vi "Trajectory_Execution_EXECUTE_REVERSE.vi"(5 "Track Width FT":dbl, 6 "RamseteEnable":bool=TRUE, 7 "Max Speed\nFT/SEC":dbl, 8 "Init":bool, 9 "Gyro Continous\n (inc counterclockwise)":dbl, 10 "Right Distance":dbl, 11 "Left Distance":dbl) -> (0 "AtReference":bool, 1 "Right Speed Target":dbl, 2 "Left Speed Target":dbl, 3 "outRAMSETE (SI)":T5={"B"=2.0, "Zeta"=0.7, "poseTolerance"={"TRANSLATION"={"X"=0.0, "Y"=0.0}, "ROTATION"={"VALUE"=0.0, "COS"=1.0, "SIN"=0.0}}, "poseError"={"TRANSLATION"={"X"=0.0, "Y"=0.0}, "ROTATION"={"VALUE"=0.0, "COS"=1.0, "SIN"=0.0}}, "Enabled"=TRUE} {"poseError"."ROTATION"."SIN" format="%13.4f"; "poseError"."ROTATION"."COS" format="%13.4f"; "poseError"."ROTATION"."VALUE" format="%13.4f"; "poseError"."TRANSLATION"."Y" format="%14.3f"; "poseError"."TRANSLATION"."X" format="%14.3f"; "poseTolerance"."ROTATION"."SIN" format="%13.4f"; "poseTolerance"."ROTATION"."COS" format="%13.4f"; "poseTolerance"."ROTATION"."VALUE" format="%13.4f"; "poseTolerance"."TRANSLATION"."Y" format="%14.3f"; "poseTolerance"."TRANSLATION"."X" format="%14.3f"; "Zeta" format="%12.3f"; "B" format="%12.3f"}, 4 "OutputTRAJ_STATE (SI)":T1={"TimeSeconds"=0.0, "Velocity"=0.0, "Acceleration"=0.0, "POSE"={"TRANSLATION"={"X"=0.0, "Y"=0.0}, "ROTATION"={"VALUE"=0.0, "COS"=1.0, "SIN"=0.0}}, "Curvature"=0.0} {"POSE"."ROTATION"."SIN" format="%13.4f"; "POSE"."ROTATION"."COS" format="%13.4f"; "POSE"."ROTATION"."VALUE" format="%13.4f"; "POSE"."TRANSLATION"."Y" format="%14.3f"; "POSE"."TRANSLATION"."X" format="%14.3f"})   [LabVIEW 2019]
uses:
  <vilib>/Rock Robotics/WPI/ThirdParty/JAS_Junk/TrajLib/TypeDef/RAMSETE.ctl
  <vilib>/Rock Robotics/WPI/ThirdParty/JAS_Junk/TrajLib/TypeDef/POSE2D.ctl
  <vilib>/Rock Robotics/WPI/ThirdParty/JAS_Junk/TrajLib/TypeDef/TRANSLATION2D.ctl
  <vilib>/Rock Robotics/WPI/ThirdParty/JAS_Junk/TrajLib/TypeDef/ROTATION2D.ctl
  <vilib>/Rock Robotics/WPI/ThirdParty/JAS_Junk/TrajLib/TypeDef/TRAJ_STATE.ctl
  <vilib>/Rock Robotics/WPI/ThirdParty/JAS_Junk/TrajLib/Conv_Feet_Meters.vi
  <vilib>/Rock Robotics/WPI/ThirdParty/JAS_Junk/TrajLib/Conv_Deg_Radians.vi
  <vilib>/Rock Robotics/WPI/ThirdParty/JAS_Junk/TrajLib/Ramsete_Execute.vi
  <vilib>/Rock Robotics/WPI/ThirdParty/JAS_Junk/TrajLib/Conv_Meters_Feet.vi
  <vilib>/Rock Robotics/WPI/ThirdParty/JAS_Junk/TrajLib/Conv_POSE2D_SI_Eng.vi
  <vilib>/Rock Robotics/WPI/ThirdParty/JAS_Junk/TrajLib/Ramsete_New_B_Z.vi
  <vilib>/Rock Robotics/WPI/ThirdParty/JAS_Junk/TrajLib/Ramsete_SetTolerance.vi
  <vilib>/Rock Robotics/WPI/ThirdParty/JAS_Junk/TrajLib/Pose2d_New.vi
  <vilib>/Rock Robotics/WPI/ThirdParty/JAS_Junk/TrajLib/Conv_AngleRadians_Heading.vi
  <vilib>/Rock Robotics/WPI/ThirdParty/JAS_Junk/TrajLib/Ramsete_SetEnabled.vi
  <vilib>/Rock Robotics/WPI/ThirdParty/JAS_Junk/TrajLib/Conv_Radians_Deg.vi
  <vilib>/Rock Robotics/WPI/ThirdParty/JAS_Junk/TrajLib/Rotation2d_CreateAngle.vi
  <vilib>/Rock Robotics/WPI/ThirdParty/JAS_Junk/TrajLib/Translation2d_Create.vi
  <vilib>/Rock Robotics/WPI/ThirdParty/JAS_Junk/TrajLib/Ramsete_Diff_DO_SI.vi
  <vilib>/Rock Robotics/WPI/ThirdParty/JAS_Junk/TrajLib/DiffWheel_Normalize.vi
  Trajectory_Execution_Globals.vi
  <vilib>/Rock Robotics/WPI/ThirdParty/JAS_Junk/TrajLib/Trajectory_Library.lvlib
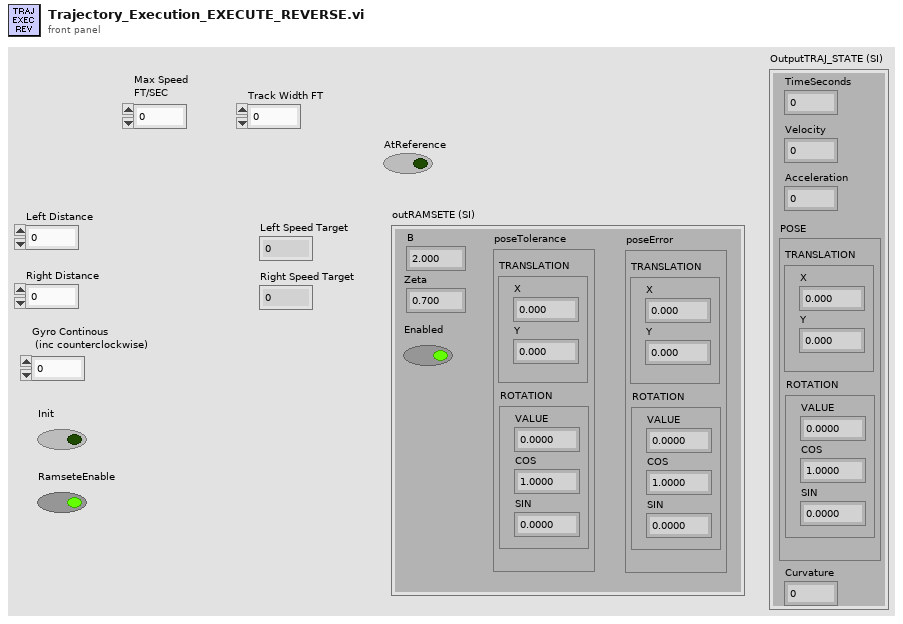
[diagram p1: front panel]
types:
  T1 = typedef "Trajectory_Library.lvlib/TRAJ_STATE.ctl" = cluster{"TimeSeconds":dbl, "Velocity":dbl, "Acceleration":dbl, "POSE":T2, "Curvature":dbl}
  T2 = typedef "Trajectory_Library.lvlib/POSE2D.ctl" = cluster{"TRANSLATION":T3, "ROTATION":T4}
  T3 = typedef "Trajectory_Library.lvlib/TRANSLATION2D.ctl" = cluster{"X":dbl, "Y":dbl}
  T4 = typedef "Trajectory_Library.lvlib/ROTATION2D.ctl" = cluster{"VALUE":dbl, "COS":dbl, "SIN":dbl}
  T5 = typedef "Trajectory_Library.lvlib/RAMSETE.ctl" = cluster{"B":dbl, "Zeta":dbl, "poseTolerance":T2, "poseError":T2, "Enabled":bool}
  T6 = typedef "Trajectory_Library.lvlib/TRAJECTORY.ctl" = cluster{"TotalTImeSecs":dbl, "States":T1[]}
  T7 = typedef "Trajectory_Library.lvlib/RAMSETE_EXE_TUNING.ctl" = cluster{"B":dbl, "Zeta":dbl, "X Tolerance M":dbl, "Y Tolerance M":dbl, "Heading Tolerance RAD":dbl, "Track Width M":dbl, "Max Speed M/S":dbl}
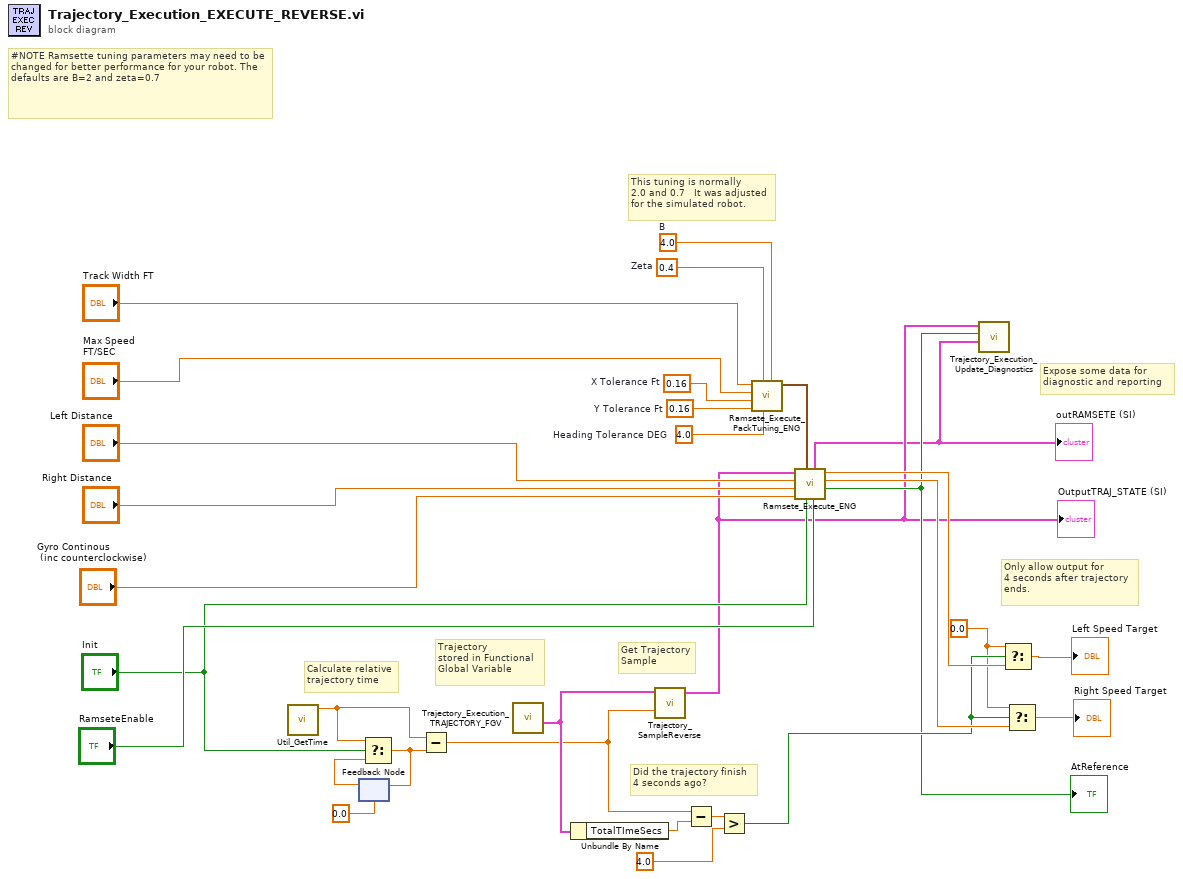
[diagram p0: block diagram]
diagram:
  w10 = 0.0 ("t")
  w25 = 0.16  # X Tolerance Ft
  w24 = 0.16  # Y Tolerance Ft
  w23 = 0.4  # Zeta
  w22 = 4.0  # Heading Tolerance DEG
  w21 = 4.0  # B
  # "This tuning is normally\n2.0 and 0.7   It was adjusted\nfor the simulated robot."
  # "Expose some data for\ndiagnostic and reporting"
  # "Did the trajectory finish\n4 seconds ago?"
  # "Get Trajectory\nSample"
  # "Trajectory\nstored in Functional\nGlobal Variable"
  # "Calculate relative\ntrajectory time"
  # "#NOTE Ramsette tuning parameters may need to be changed for better performance for your robot. The defaults are B=2 and zeta=0.7"
  # "Only allow output for\n4 seconds after trajectory\nends."
  n1 = call <vilib>:"Util_GetTime.vi"() -> ("FPGA_Time_Seconds"=w4:dbl)  [unwired: 10 in, 1 out]
  n2 = feedback #1(0.0 ("TIME")) -> (w6:dbl)
  n3 = Select(t=w4, s="Init", f=w6) -> (s? t:f=w7:dbl)
  n4 = feedback-in #1(w7) -> ()
  n5 = Subtract(x=w4, y=w7) -> (x-y=w28:dbl)
  n6 = call "Trajectory_Execution_TRAJECTORY_FGV.vi"() -> ("outTRAJECTORY"=w30:T6)  [unwired: 11 in]
  n7 = Unbundle By Name(w30) -> ("TotalTImeSecs"=w29:dbl)
  n8 = call <vilib>:"Trajectory_SampleReverse.vi"("Time"=w28, "InputTRAJECTORY"=w30) -> ("OutputTRAJ_STATE"=w2:T1)  [unwired: 9 in]
  "OutputTRAJ_STATE (SI)" <- w2
  n9 = Subtract(x=w28, y=w29) -> (x-y=w27:dbl)
  n10 = Greater?(x=w27, y=4.0) -> (0:w11:bool)
  n11 = call <vilib>:"Ramsete_Execute_PackTuning_ENG.vi"("B"=w21, "Heading Tolerance DEG"=w22, "Zeta"=w23, "Y Tolerance Ft"=w24, "X Tolerance Ft"=w25, "Max Speed Ft/S"="Max Speed\nFT/SEC", "Track Width Ft"="Track Width FT") -> ("RAMSETE_EXE_TUNING"=w20:T7)  [unwired: 4 in]
  n12 = call <vilib>:"Ramsete_Execute_ENG.vi"("Enabled"="RamseteEnable", "Reset"="Init", "RAMSETE_EXE_TUNING"=w20, "Gyro-Deg\n(Inc counterclockwise)"="Gyro Continous\n (inc counterclockwise)", "RightDist-Ft"="Right Distance", "LeftDist-Ft"="Left Distance", "TRAJ_STATE  SI"=w2) -> ("AtReference"=w3:bool, "Right Speed Dmd Ft/S"=w13:dbl, "Left Speed Dmd Ft/S"=w12:dbl, "outRAMSETE"=w1:T5)  [unwired: 1 out]
  "AtReference" <- w3
  "outRAMSETE (SI)" <- w1
  n13 = call "Trajectory_Execution_Update_Diagnostics.vi"("outRAMSETE (SI)"=w1, "AtReference"=w3, "OutputTRAJ_STATE (SI)"=w2) -> ()  [unwired: 9 in]
  n14 = Select(t=w10, s=w11, f=w12) -> (s? t:f=→"Left Speed Target":dbl)
  n15 = Select(t=w10, s=w11, f=w13) -> (s? t:f=→"Right Speed Target":dbl)
